vi "Nichtlineares Pendelmodell Sub.vi"(0 "Kraft (N)":dbl, 1 "Position_t0":dbl, 2 "Winkel_t0":dbl, 3 "Winkelg._t0":dbl) -> (7 "Position":dbl, 8 "Geschwindigkeit":dbl, 9 "Winkel":dbl, 10 "Winkelgesch":dbl)   [LabVIEW 2014]
uses:
  <vilib>/Simulation/Implementation/Shared/SIMSCR Execution Mode.ctl
  <vilib>/Simulation/Scripting/Companion Diagram/SimConfigNode/SimParams.ctl
  <vilib>/Simulation/Scripting/Companion Diagram/SimConfigNode/_simSolvers.ctl
  <vilib>/Simulation/Param Hierarchy/Typedefs/SIMPH Param Control Actions.ctl
  <vilib>/Simulation/Implementation/Shared/SIM limit type.ctl
  <vilib>/Simulation/Implementation/Shared/NILVSim_ParamChanged.vi
  <vilib>/Simulation/Implementation/Shared/NILVSIM_BeginStep.vi
  <vilib>/Simulation/ContinuousLinear/Implementation/NILVSim Integrator new.llb/SIM Integrator distributor (scalar).vi
  <vilib>/Simulation/ContinuousLinear/Implementation/NILVSim Integrator new.llb/SIM Integrator collector (scalar).vi
  <vilib>/Simulation/Implementation/Shared/NILVSim_Manager.vi
  <vilib>/Utility/error.llb/Clear Errors.vi
  <vilib>/Simulation/Implementation/Shared/NILVSim_FinalizeModel.vi
  <vilib>/Simulation/Implementation/Shared/SIM Unbundle Sim Info.vi
  <vilib>/Simulation/Implementation/Shared/SIMSH Read Queue.vi
  <vilib>/Simulation/Implementation/Shared/NILVSim_Initialize.vi
  <vilib>/Simulation/Utility/Implementation/NILVSim Get Time and IsAcceptedStep.vi
  <vilib>/Simulation/Implementation/Shared/NILVSim_GetModelError.vi
  <vilib>/Simulation/Implementation/Shared/SIM SimErrorHandler.vi
  <vilib>/Simulation/Implementation/Shared/SIM Bundle Sim Info.vi
  <vilib>/Simulation/Scripting/Companion Diagram/SimConfigNode/SimDog.xnode
  <vilib>/Simulation/ContinuousLinear/Implementation/NILVSim Integrator new.llb/SIM Integrator (scalar).vi
  <vilib>/Simulation/Implementation/XNodeFramework/SimXNode/SimX.xnode
  <vilib>/Simulation/Implementation/Shared/NI_SIM_Implementation.lvlib
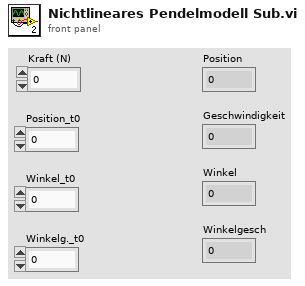
[diagram p1: front panel]
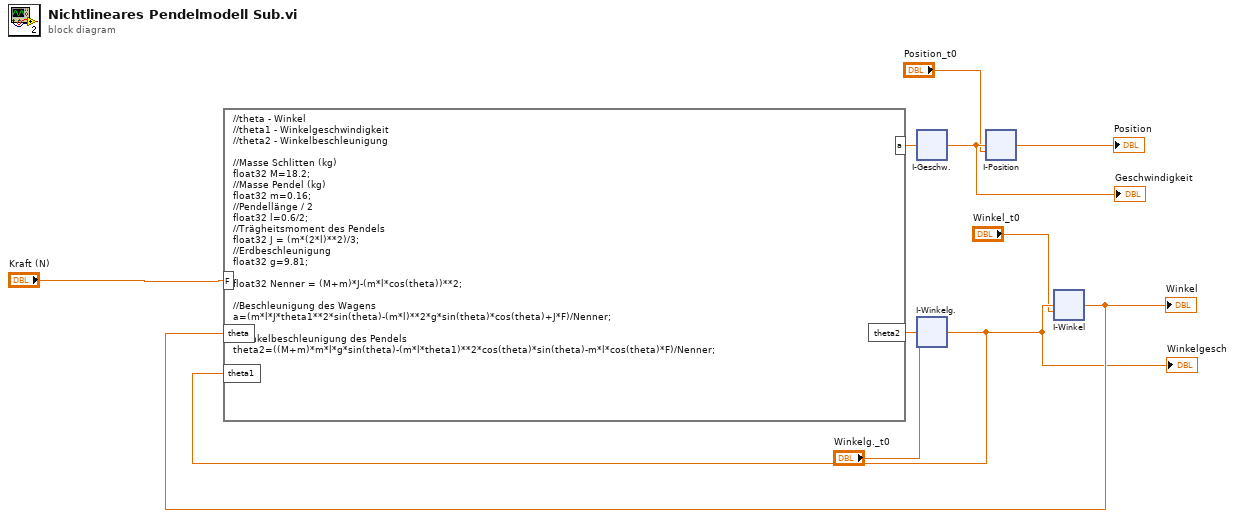
[diagram p0: block diagram]
diagram:
  n1 = formula code="//theta - Winkel\n//theta1 - Winkelgeschwindigkeit\n//theta2 - Winkelbeschleunigung\n\n//Masse Schlitten (kg)\nfloat32 M=18.2;\n//Masse Pendel (kg)\nfloat32 m=0.16;\n//Pendellänge / 2\nfloat32 l=0.6/2;\n//Trägheitsmoment des Pendels\nfloat32 J = (m*(2*l)**2)/3;\n//Erdbeschleunigung\nfloat32 g=9.81;\n\nfloat32 Nenner = (M+m)*J-(m*l*cos(theta))**2;\n\n//Beschleunigung des Wagens\na=(m*l*J*theta1**2*sin(theta)-(m*l)**2*g*sin(theta)*cos(theta)+J*F)/Nenner;\n\n//Winkelbeschleunigung des Pendels\ntheta2=((M+m)*m*l*g*sin(theta)-(m*l*theta1)**2*cos(theta)*sin(theta)-m*l*cos(theta)*F)/Nenner;" ("Formelknoten")("theta"=w10, "theta1"=w8, "F"="Kraft (N)") -> ("a"=w3:dbl, "theta2"=w4:dbl)
  n2 = xnode "I-Geschw."("input"=w3) -> ("output"=w7:dbl)  [unwired: 9 in, 2 out]
  "Geschwindigkeit" <- w7
  n3 = xnode "I-Winkelg."("input"=w4, "initial condition"="Winkelg._t0") -> ("output"=w8:dbl)  [unwired: 8 in, 2 out]
  "Winkelgesch" <- w8
  n4 = xnode "I-Position"("input"=w7, "initial condition"="Position_t0") -> ("output"=→"Position":dbl)  [unwired: 8 in, 2 out]
  n5 = xnode "I-Winkel"("input"=w8, "initial condition"="Winkel_t0") -> ("output"=w10:dbl)  [unwired: 8 in, 2 out]
  "Winkel" <- w10
